vi "Clean Tree.vi"(11 "TreeControl in":refnum<vi>) -> (0 "error out":errorcluster)   [LabVIEW 2020, in "Panther Dashboard.lvlib"]
uses:
  Panther Dashboard.lvlib
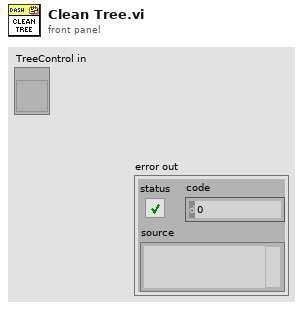
[diagram p1: front panel]
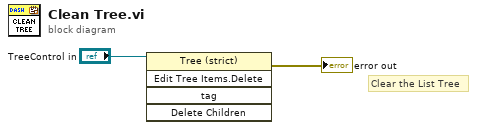
[diagram p0: block diagram]
diagram:
  # "Clear the List Tree"
  n1 = invoke class="Tree (strict)" method="Edit Tree Items.Delete"(reference="TreeControl in") -> (error out=→"error out":errorcluster)  [unwired: 4 in, 4 out]
